vi "Working With Numeric Arrays.vi"() -> ()   [LabVIEW 2015]
uses:
  <vilib>/NI/JSON Support for LabVIEW/JSON Data Classes/JSON Array/New JSON Array (Numeric).vi
  <vilib>/NI/JSON Support for LabVIEW/JSON Data Classes/JSON Array/Get Array Values as Numerics.vi
  <vilib>/NI/JSON Support for LabVIEW/JSON Data Classes/JSON Array/Array Max & Min Numeric Value.vi
  <vilib>/NI/JSON Support for LabVIEW/JSON Data Classes/JSON Numeric/New JSON Numeric.vi
  <vilib>/NI/JSON Support for LabVIEW/JSON Data Classes/JSON Array/Replace Array Subset (Single).vi
  <vilib>/NI/JSON Support for LabVIEW/JSON Data Classes/JSON Helper/JSON Helper.lvclass
  <vilib>/NI/JSON Support for LabVIEW/JSON Data Classes/JSON Array/JSON Array.lvclass
  <vilib>/NI/JSON Support for LabVIEW/JSON Data Classes/JSON Numeric/JSON Numeric.lvclass
panel:
  out "split 2-end":dbl[](array[numeric])
  out "split 0-1":dbl[](array[numeric])
  out "search for 10":i32
  out "reversed":dbl[](array[numeric])
  out "replace 3 with 10":dbl[](array[numeric])
  out "initial values":dbl[](array[numeric])
  out "subset 1,3":dbl[](array[numeric])
  out "sorted values":dbl[](array[numeric])
  out "min value":dbl
  out "max value":dbl
  out "min index":i32
  out "max index":i32
  out "size(s)":i32
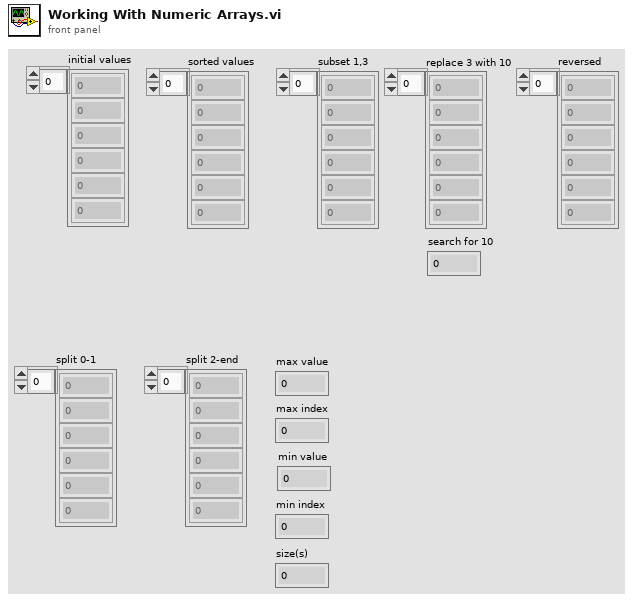
[diagram p1: front panel]
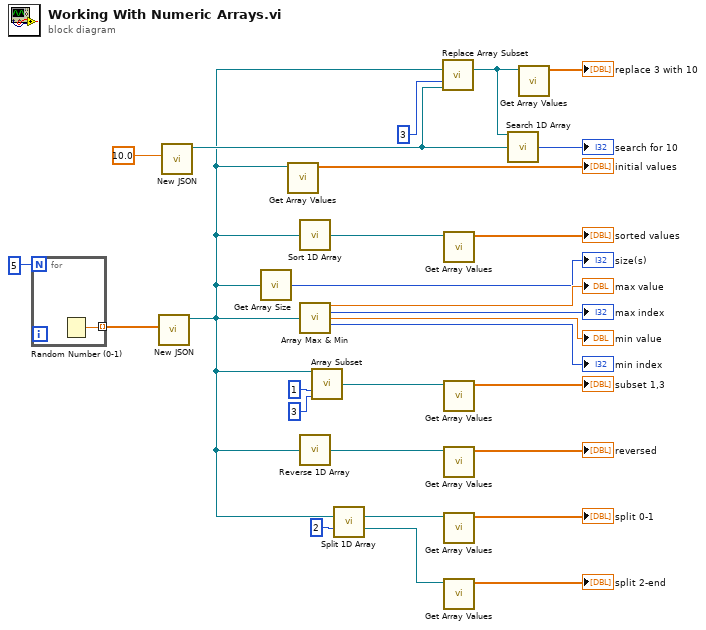
[diagram p0: block diagram]
diagram:
  n1 = for {
    N: 5 -> [_]
    tunnel: [w29] -> w28 mode=indexing
    n2 = Random Number (0-1)() -> (number: 0 to 1=w29:dbl)
  }
  n3 = call-poly <vilib>:"New JSON.vi"("Numeric Array"=w28) -> ("JSON Array out"=w6:refnum<class "JSON Array.lvclass">)  [unwired: 9 in, 1 out]
  n4 = call-poly <vilib>:"New JSON.vi"("value"=10.0) -> ("JSON String out"=w8:refnum<class "JSON Numeric.lvclass">)  [unwired: 9 in, 1 out]
  n5 = call <vilib>:"Get Array Size.vi"("JSON Array in"=w6) -> ("size(s)"=→"size(s)":i32)
  n6 = call-poly <vilib>:"Get Array Values.vi"("JSON Array in"=w6) -> ("values"=→"initial values":dbl[])  [unwired: 9 in, 1 out]
  n7 = call <vilib>:"Sort 1D Array.vi"("JSON Array"=w6) -> ("sorted JSON Array"=w21:refnum<class "JSON Array.lvclass">)  [unwired: 13 in, 1 out]
  n8 = call-poly <vilib>:"Array Max & Min.vi"("JSON Array"=w6) -> ("max value"=→"max value":dbl, "max index"=→"max index":i32, "min value"=→"min value":dbl, "min index"=→"min index":i32)  [unwired: 10 in, 1 out]
  n9 = call <vilib>:"Reverse 1D Array.vi"("JSON Array"=w6) -> ("reversed JSON Array"=w10:refnum<class "JSON Array.lvclass">)  [unwired: 14 in]
  n10 = call <vilib>:"Array Subset.vi"("JSON Array"=w6, "index"=1, "length"=3) -> ("JSON Array out"=w16:refnum<class "JSON Array.lvclass">)  [unwired: 12 in]
  n11 = call <vilib>:"Split 1D Array.vi"("JSON Array"=w6, "index"=2) -> ("first subarray"=w2:refnum<class "JSON Array.lvclass">, "second subarray"=w1:refnum<class "JSON Array.lvclass">)  [unwired: 12 in]
  n12 = call-poly <vilib>:"Replace Array Subset.vi"("JSON Array"=w6, "index"=3, "new element/subarray"=w8) -> ("output JSON Array"=w9:refnum<class "JSON Array.lvclass">)  [unwired: 12 in]
  n13 = call-poly <vilib>:"Get Array Values.vi"("JSON Array in"=w21) -> ("values"=→"sorted values":dbl[])  [unwired: 9 in, 1 out]
  n14 = call-poly <vilib>:"Get Array Values.vi"("JSON Array in"=w16) -> ("values"=→"subset 1,3":dbl[])  [unwired: 9 in, 1 out]
  n15 = call-poly <vilib>:"Get Array Values.vi"("JSON Array in"=w10) -> ("values"=→"reversed":dbl[])  [unwired: 9 in, 1 out]
  n16 = call-poly <vilib>:"Get Array Values.vi"("JSON Array in"=w2) -> ("values"=→"split 0-1":dbl[])  [unwired: 9 in, 1 out]
  n17 = call-poly <vilib>:"Get Array Values.vi"("JSON Array in"=w1) -> ("values"=→"split 2-end":dbl[])  [unwired: 9 in, 1 out]
  n18 = call <vilib>:"Search 1D Array.vi"("JSON Array"=w9, "element"=w8) -> ("index of element"=→"search for 10":i32)  [unwired: 13 in]
  n19 = call-poly <vilib>:"Get Array Values.vi"("JSON Array in"=w9) -> ("values"=→"replace 3 with 10":dbl[])  [unwired: 9 in, 1 out]
